vi "Get Row Data.vi"(8 "error in (no error)":errorcluster, 10 "Row Index":i32, 11 "SLL Table in":refnum<class "SLL Table.lvclass">) -> (0 "error out":errorcluster, 2 "Row Map":map{string, string}(c390), 3 "SLL Table out":refnum<class "SLL Table.lvclass">)   [LabVIEW 2019, in "SLL Table.lvclass"]
doc: "Returns the row data as a map"
uses:
  SLL Table.lvclass
  SLL Table.lvclass/SLL Table.ctl
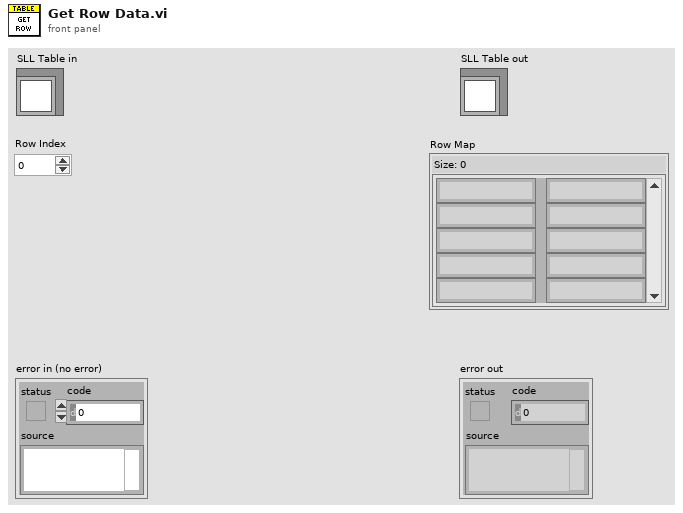
[diagram p1: front panel]
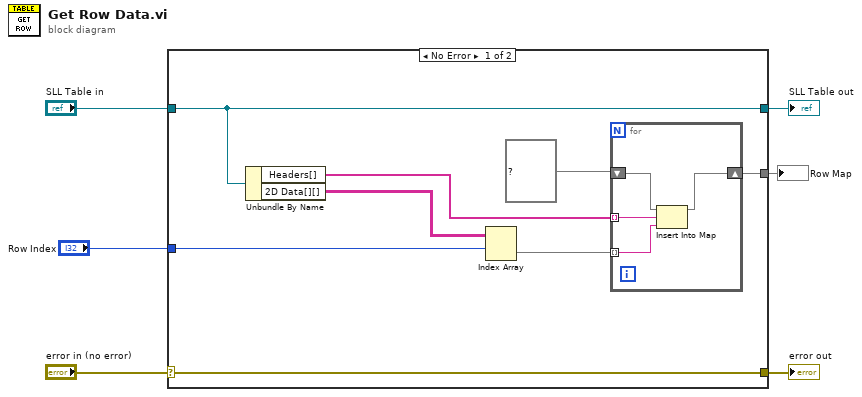
[diagram p0: block diagram]
diagram:
  n1 = case shown="No Error" "error in (no error)" {
    selector: "error in (no error)" -> [w14 w20]
    tunnel: [w14 w20] -> w5
    tunnel: [w13 w19] -> w3
    tunnel: "SLL Table in" -> [w13 w19]
    tunnel: "Row Index" -> [w12 _]
    tunnel: [w7 _] -> w1
    frame No Error {
      n2 = Unbundle By Name(w13) -> ("Headers[]"=w11:string[], "2D Data[][]"=w9:string[][])
      n3 = Index Array(array=w9, index (row)=w12) -> (element=w10:string[])  [unwired: 1 in]
      n4 = for {
        tunnel: w11 -> [w18] mode=indexing
        tunnel: w10 -> [w17] mode=indexing
        shift-right: [w15] -> w7
        shift-left: map{string, string} {} ("map") -> [w16]
        n5 = Insert Into Map(map in=w16, key=w18, value=w17) -> (map out=w15:map{string, string})  [unwired: 2 out]
      }
    }
    frame Error {
    }
  }
  "error out" <- w5
  "SLL Table out" <- w3
  "Row Map" <- w1
